vi "Start.vi"(8 "error in (no error)":errorcluster, 10 "Message in":refnum<class "StartMessage.lvclass">, 11 "ImageStack in":refnum<class "ImageStack.lvclass">) -> (0 "error out":errorcluster, 3 "ImageStack out":refnum<class "ImageStack.lvclass">)   [LabVIEW 2012, in "ImageStack.lvclass"]
doc: "This member function is called when the statemachine in the run.vi receives an 'start' command. It relays the message to all observers of the component.\n\nOverride this member function in your derived class if you need additional start functionality (but don't forget to call the parent method)."
uses:
  ImageStack.lvclass
  <vilib>/Distrio/Murmex/StartMessage/StartMessage.lvclass
  <vilib>/Distrio/Murmex/StartMessage/run mode enum.ctl
  ImageStack.lvclass/ImageStack.ctl
  <vilib>/Distrio/Murmex/Murmex/Murmex.lvclass
panel:
  # "This member function is called when the statemachine in the run.vi receives an 'start' command. It relays the message to all observers of the component.\n\nOverride this member function in your derived class if you need additional start functionality (but don't forget to call the parent method)."
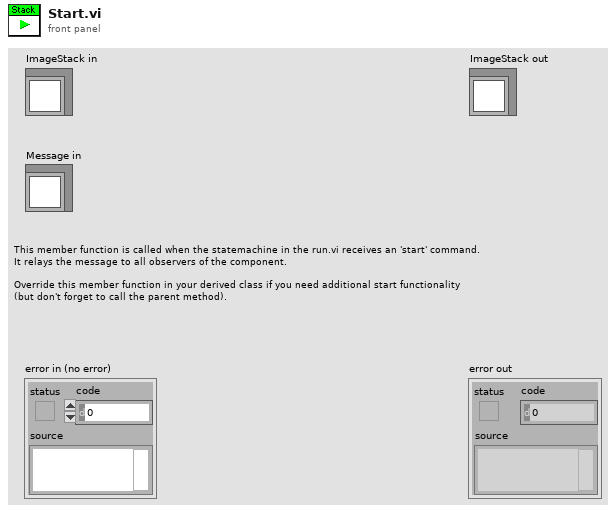
[diagram p1: front panel]
types:
  T1 = typedef "Murmex.lvlib/StartMessage.lvclass/run mode enum.ctl" = enum16{"infinite", "finite"}
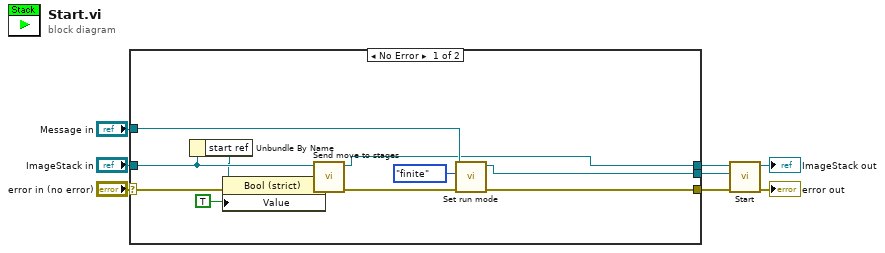
[diagram p0: block diagram]
diagram:
  n1 = case shown="No Error" "error in (no error)" {
    selector: "error in (no error)" -> [w11 w22]
    tunnel: [w18 w22] -> w5
    tunnel: [w15 w21] -> w7
    tunnel: "Message in" -> [w19 w20]
    tunnel: [w14 w20] -> w6
    tunnel: "ImageStack in" -> [w13 w21]
    frame No Error {
      n2 = Unbundle By Name(w13) -> ("start ref"=w12:refnum<vi>)
      n3 = property class="Bool (strict)"(reference=w12, error in=w11, "Value"=TRUE) -> (error out=w10:errorcluster)  [unwired: 1 out]
      n4 = call-dynamic "Send move to stages.vi"("error in (no error)"=w10, "ImageStack in"=w13) -> ("error out"=w16:errorcluster, "ImageStack out"=w15:refnum<class "ImageStack.lvclass">)  [unwired: 8 in]
      n5 = call <vilib>:"Set run mode.vi"("error in (no error)"=w16, "run mode"=run_mode_enum."finite", "StartMessage in"=w19) -> ("error out"=w18:errorcluster, "StartMessage out"=w14:refnum<class "StartMessage.lvclass">)  [unwired: 7 in]
    }
    frame Error {
    }
  }
  n6 = call-parent "Start.vi"("error in (no error)"=w5, "Message in"=w6, "Murmex in"=w7) -> ("error out"=→"error out":errorcluster, "Murmex out"=→"ImageStack out":refnum<class "ImageStack.lvclass">)  [unwired: 7 in]
